vi "niRFUtil WFM Trace Detector.vi"(0 "Real Waveform In (dBm)":T4 {"y" min=0 max=127 format="%.2f"; "dx" format="%^.2e"; "x0" format="%^.2e"}, 5 "Number of Points":T1=1001, 7 "Detector Type":T6=enum."Peak", 11 "error in (no error)":errorcluster, 12 "Averaging Enabled":T3, 13 "Averaging Type":T2) -> (4 "Real Waveform Out (dBm)":T4 {"y" min=0 max=127 format="%.2f"; "dx" format="%^.2e"; "x0" format="%^.2e"}, 6 "Bins per Bucket":i32[](array[numeric]), 15 "error out":errorcluster)   [LabVIEW 2015, in "niRFUtil.lvlib"]
uses:
  niRFUtil.lvlib
  Includes/niRFUtil INC Detector Type.ctl
  Includes/niRFUtil INC Real Waveform.ctl
  Includes/niRFUtil INC Real Array.ctl
  Includes/niRFUtil INC Averaging Enabled.ctl
  Includes/niRFUtil INC Averaging Type (Freq Domain).ctl
  Includes/niRFUtil INC Detector Points.ctl
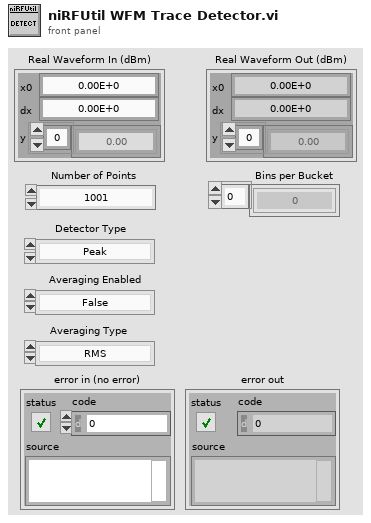
[diagram p1: front panel]
types:
  T1 = typedef "niRFUtil.lvlib/niRFUtil INC Detector Points.ctl" = i32
  T2 = typedef "niRFUtil.lvlib/niRFUtil INC Averaging Type (Freq Domain).ctl" = enum16{"RMS", "Log", "Scalar", "Max", "Min", "Vector"}
  T3 = typedef "niRFUtil.lvlib/niRFUtil INC Averaging Enabled.ctl" = enum16{"False", "True"}
  T4 = typedef "niRFUtil.lvlib/niRFUtil INC Real Waveform.ctl" = cluster{"x0":dbl, "dx":dbl, "y":T5}
  T5 = typedef "niRFUtil.lvlib/niRFUtil INC Real Array.ctl" = sgl[]
  T6 = typedef "niRFUtil.lvlib/niRFUtil INC Detector Type.ctl" = enum16{"Sample", "Normal", "Peak", "Negative Peak", "Average RMS", "Average Voltage", "Average Log"}
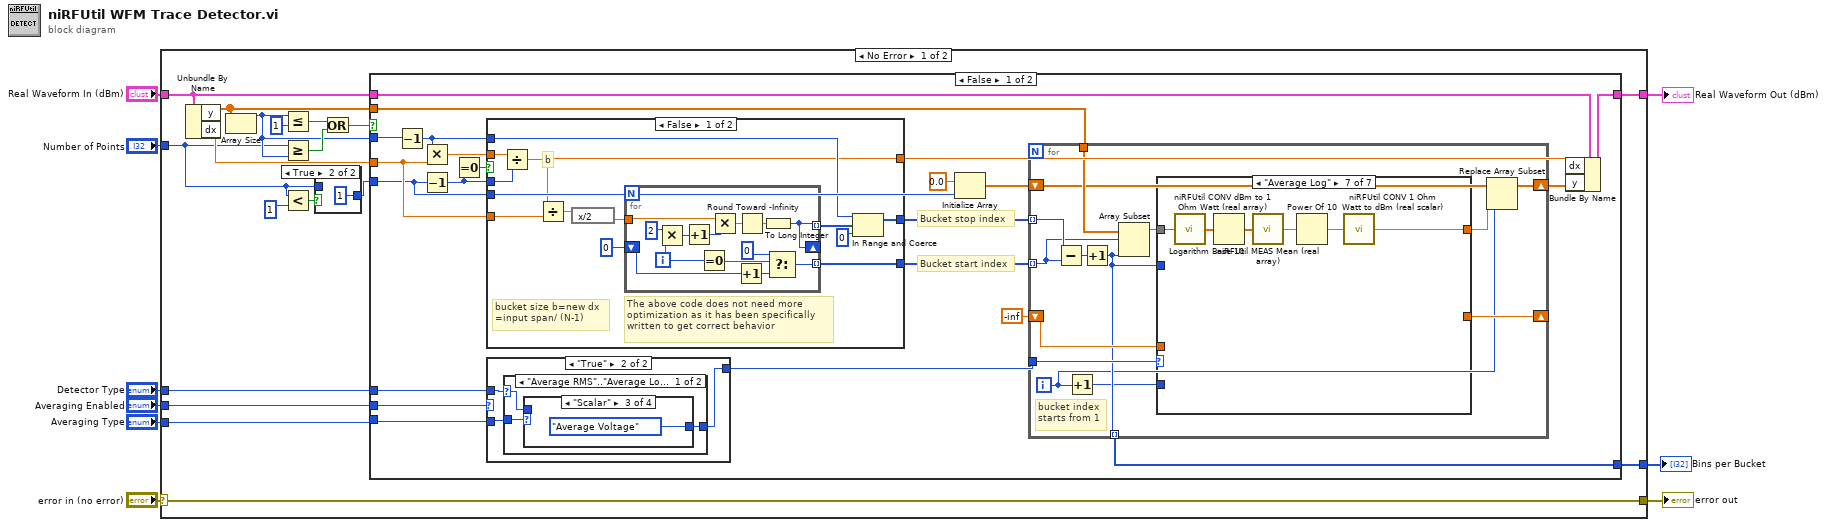
[diagram p0: block diagram]
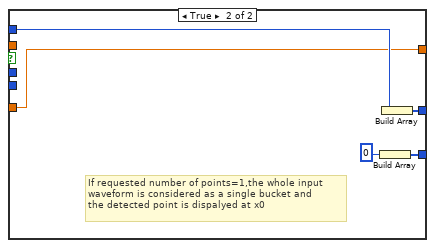
[diagram p3: hidden frame]
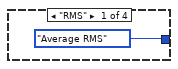
[diagram p5: hidden frame]
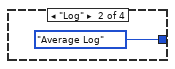
[diagram p6: hidden frame]
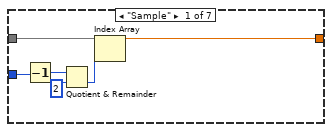
[diagram p9: hidden frame]
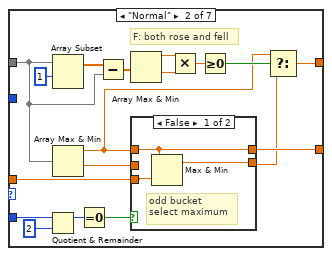
[diagram p10: hidden frame]
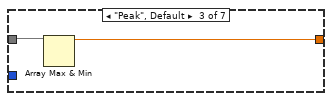
[diagram p12: hidden frame]
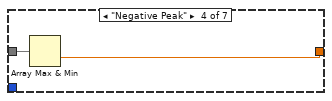
[diagram p13: hidden frame]
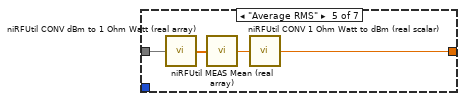
[diagram p14: hidden frame]
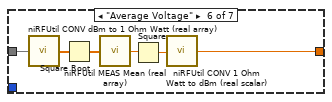
[diagram p15: hidden frame]
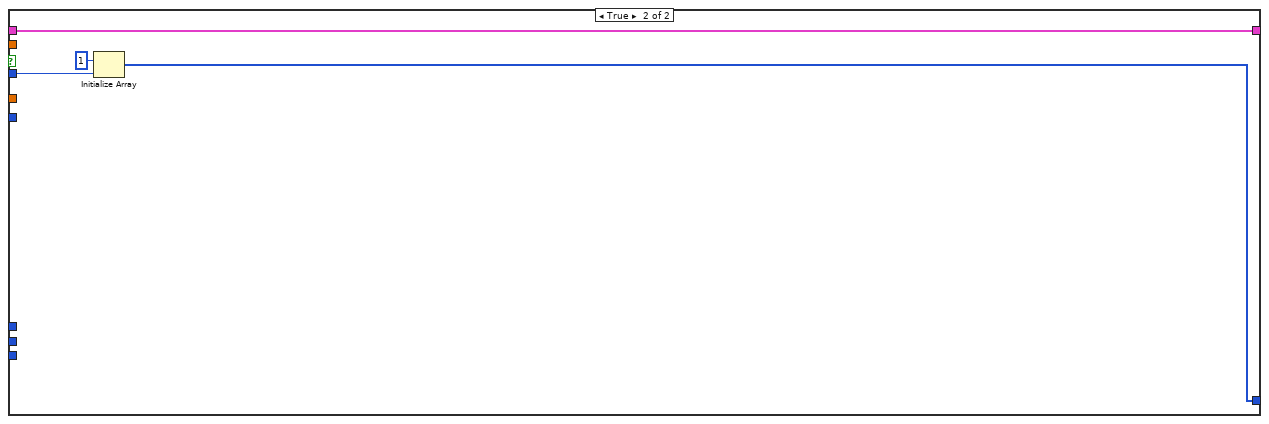
[diagram p16: hidden frame]
diagram:
  n1 = case shown="No Error" "error in (no error)" {
    selector: "error in (no error)" -> [w21 w161]
    tunnel: "Detector Type" -> [w27 _]
    tunnel: "Number of Points" -> [w10 _]
    tunnel: [w26 _] -> w8
    tunnel: [w25 w162] -> w7
    tunnel: "Real Waveform In (dBm)" -> [w24 w162]
    tunnel: "Averaging Enabled" -> [w23 _]
    tunnel: "Averaging Type" -> [w22 _]
    tunnel: [w21 w161] -> w2
    frame No Error {
      n2 = Unbundle By Name(w24) -> ("y"=w19:T5, "dx"=w20:dbl)
      n3 = Array Size(array=w19) -> (size(s)=w14:i32)
      n4 = Less Or Equal?(x=w14, y=1) -> (x <= y?=w17:bool)
      n5 = Greater Or Equal?(x=w10, y=w14) -> (x >= y?=w15:bool)
      n6 = Less?(x=w10, y=T1 1) -> (x < y?=w12:bool)
      n7 = case shown="True" w12 {
        tunnel: w10 -> [w28 _]
        tunnel: [w28 T1 1 ("Number of Points")] -> w11
        frame False {
        }
        frame True {
        }
      }
      n8 = Or(x=w17, y=w15) -> (x .or. y?=w16:bool)
      n9 = case shown="False" w16 {
        tunnel: w27 -> [w39 _]
        tunnel: [w49 w160] -> w25
        tunnel: w20 -> [w42 _]
        tunnel: [w46 w157] -> w26
        tunnel: w24 -> [w44 w160]
        tunnel: w19 -> [w45 _]
        tunnel: w14 -> [w41 w158]
        tunnel: w23 -> [w38 _]
        tunnel: w22 -> [w37 _]
        tunnel: w11 -> [w30 _]
        frame False {
          # "Bucket start index"
          # "Bucket stop index"
          n10 = Decrement(x=w41) -> (x-1=w43:i32)
          n11 = Multiply(x=w43, y=w42) -> (x*y=w51:dbl)
          n12 = Decrement(x=w30) -> (x-1=w32:T1)
          n13 = Equal To 0?(x=w32) -> (x = 0?=w33:bool)
          n14 = case shown="False" w33 {
            tunnel: w51 -> [w64 _]
            tunnel: [w62 w81] -> w48
            tunnel: [w61 w78] -> w47
            tunnel: w43 -> [w56 w82]
            tunnel: w42 -> [w55 w80]
            tunnel: [w54 w80] -> w40
            tunnel: w32 -> [w52 _]
            tunnel: w30 -> [w53 _]
            frame False {
              # "The above code does not need more \noptimization as it has been specifically \nwritten to get correct behavior"
              # "b"
              # "bucket size b=new dx\n=input span/ (N-1)"
              n15 = Divide(x=w64, y=w52) -> (x/y=w54:dbl)
              n16 = Divide(x=w54, y=w55) -> (x/y=w59:dbl)
              n17 = expression code="x/2"(w59) -> (w58:dbl)
              n18 = for {
                N: w53 -> [_]
                tunnel: w58 -> [w74]
                shift-right: [w65] -> _
                shift-left: 0 -> [w69]
                tunnel: [w67] -> w61 mode=indexing
                tunnel: [w65] -> w63 mode=indexing
                i -> [w72]
                n19 = Multiply(x=2 ("y"), y=w72) -> (x*y=w76:i32)
                n20 = Increment(x=w76) -> (x+1=w75:i32)
                n21 = Equal To 0?(x=w72) -> (x = 0?=w71:bool)
                n22 = Multiply(x=w74, y=w75) -> (x*y=w73:dbl)
                n23 = Increment(x=w69) -> (x+1=w68:i32)
                n24 = Round Toward -Infinity(1:w73) -> (0:w66:dbl)
                n25 = To Long Integer(number=w66) -> (32bit integer=w65:i32)
                n26 = Select(t=0 ("y"), s=w71, f=w68) -> (s? t:f=w67:i32)
              }
              n27 = In Range and Coerce(upper limit=w56, x=w63, lower limit=0) -> (coerced(x)=w62:i32[])  [unwired: 1 out]
            }
            frame True {
              # "If requested number of points=1,the whole input\nwaveform is considered as a single bucket and \nthe detected point is dispalyed at x0"
              n28 = Build Array(0 ("y")) -> (w78:i32[])
              n29 = Build Array(w82) -> (w81:i32[])
            }
          }
          n30 = case shown="\"True\"" w38 {
            tunnel: w39 -> [w83 w86]
            tunnel: [w83 w85] -> w36
            tunnel: w37 -> [_ w84]
            frame "False", Default {
            }
            frame "True" {
              n31 = case shown="\"Average RMS\"..\"Average Log\"" w86 {
                selector: w86 -> [w87 w94]
                tunnel: [w88 w94] -> w85
                tunnel: w84 -> [w89 _]
                frame "Average RMS".."Average Log" {
                  n32 = case shown="\"Scalar\"" w89 {
                    tunnel: [niRFUtil_INC_Detector_Type."Average RMS" ("Detector Type") niRFUtil_INC_Detector_Type."Average Log" ("Detector Type") niRFUtil_INC_Detector_Type."Average Voltage" ("Detector Type") w93] -> w88
                    tunnel: w87 -> [_ _ _ w93]
                    frame "RMS" {
                    }
                    frame "Log" {
                    }
                    frame "Scalar" {
                    }
                    frame Default {
                    }
                  }
                }
                frame Default {
                }
              }
            }
          }
          n33 = Initialize Array(sgl 0.0 ("element"), w30) -> (w34:sgl[])
          n34 = for {
            tunnel: w45 -> [w108]
            tunnel: w47 -> [w106] mode=indexing
            tunnel: w48 -> [w107] mode=indexing
            tunnel: w36 -> [w104]
            shift-right: [w95] -> w35
            shift-left: w34 -> [w96]
            shift-right: [w102] -> _
            shift-left: sgl -inf -> [w101]
            tunnel: [w100] -> w46 mode=indexing
            i -> [w98]
            # "bucket index\nstarts from 1"
            n35 = Subtract(x=w107, y=w106) -> (x-y=w105:i32)
            n36 = Increment(x=w98) -> (x+1=w99:i32)
            n37 = Increment(x=w105) -> (x+1=w100:i32)
            n38 = Array Subset(array=w108, index=w106, length=w100) -> (w103:T5)
            n39 = case shown="\"Average Log\"" w104 {
              tunnel: w103 -> [w114 w116 w139 w141 w145 w150 w156]
              tunnel: [w113 w130 w138 w140 w144 w147 w151] -> w97
              tunnel: w99 -> [_ w129 _ _ _ _ _]
              tunnel: [_ w126 _ _ _ _ _] -> w102
              tunnel: w101 -> [_ w125 _ _ _ _ _]
              tunnel: w100 -> [w109 _ _ _ _ _ _]
              frame "Sample" {
                n40 = Decrement(x=w109) -> (x-1=w112:i32)
                n41 = Quotient & Remainder(x=w112, y=2) -> (floor(x/y)=w110:i32)  [unwired: 1 out]
                n42 = Index Array(array=w114, index=w110) -> (element=w113:sgl)
              }
              frame "Normal" {
                # "F: both rose and fell"
                n43 = Quotient & Remainder(x=w129, y=2) -> (x-y*floor(x/y)=w127:i32)  [unwired: 1 out]
                n44 = Array Subset(array=w116, index=1) -> (w117:T5)  [unwired: 1 in]
                n45 = Array Max & Min(array=w116) -> (max value=w119:sgl, min value=w118:sgl)  [unwired: 2 out]
                n46 = Equal To 0?(x=w127) -> (x = 0?=w115:bool)
                n47 = Subtract(x=w117, y=w116) -> (x-y=w131:T5)
                n48 = Array Max & Min(array=w131) -> (max value=w124:sgl, min value=w123:sgl)  [unwired: 2 out]
                n49 = case shown="False" w115 {
                  tunnel: [w134 w136] -> w120
                  tunnel: [w133 w137] -> w126
                  tunnel: w125 -> [w135 _]
                  tunnel: w119 -> [w133 w137]
                  tunnel: w118 -> [_ w136]
                  frame False {
                    # "odd bucket \nselect maximum"
                    n50 = Max & Min(x=w133, y=w135) -> (max(x,y)=w134:sgl)  [unwired: 1 out]
                  }
                  frame True {
                    # "even bucket \nselect minimum"
                  }
                }
                n51 = Multiply(x=w124, y=w123) -> (x*y=w122:sgl)
                n52 = Greater Or Equal To 0?(x=w122) -> (x >= 0?=w121:bool)
                n53 = Select(t=w119, s=w121, f=w120) -> (s? t:f=w130:sgl)
              }
              frame "Peak", Default {
                n54 = Array Max & Min(array=w139) -> (max value=w138:sgl)  [unwired: 3 out]
              }
              frame "Negative Peak" {
                n55 = Array Max & Min(array=w141) -> (min value=w140:sgl)  [unwired: 3 out]
              }
              frame "Average RMS" {
                n56 = call "niRFUtil CONV dBm to 1 Ohm Watt (real array).vi"("Real Array (dBm)"=w145) -> ("Real Array (W)"=w143:T5)  [unwired: 14 in]
                n57 = call "niRFUtil MEAS Mean (real array).vi"("Real Array"=w143) -> ("Mean"=w142:sgl)  [unwired: 14 in]
                n58 = call "niRFUtil CONV 1 Ohm Watt to dBm (real scalar).vi"("Real Scalar (W)"=w142) -> ("Real Scalar (dBm)"=w144:sgl)  [unwired: 14 in]
              }
              frame "Average Voltage" {
                n59 = call "niRFUtil CONV dBm to 1 Ohm Watt (real array).vi"("Real Array (dBm)"=w150) -> ("Real Array (W)"=w149:T5)  [unwired: 14 in]
                n60 = Square Root(x=w149) -> ()  [unwired: 1 out]
                n61 = call "niRFUtil MEAS Mean (real array).vi"("Real Array"=w149) -> ("Mean"=w146:sgl)  [unwired: 14 in]
                n62 = Square(x=w146) -> (x^2=w148:sgl)
                n63 = call "niRFUtil CONV 1 Ohm Watt to dBm (real scalar).vi"("Real Scalar (W)"=w148) -> ("Real Scalar (dBm)"=w147:sgl)  [unwired: 14 in]
              }
              frame "Average Log" {
                n64 = call "niRFUtil CONV dBm to 1 Ohm Watt (real array).vi"("Real Array (dBm)"=w156) -> ("Real Array (W)"=w155:T5)  [unwired: 14 in]
                n65 = Logarithm Base 10(1:w155) -> (0:w154:T5)
                n66 = call "niRFUtil MEAS Mean (real array).vi"("Real Array"=w154) -> ("Mean"=w153:sgl)  [unwired: 14 in]
                n67 = Power Of 10(x=w153) -> (10^x=w152:sgl)
                n68 = call "niRFUtil CONV 1 Ohm Watt to dBm (real scalar).vi"("Real Scalar (W)"=w152) -> ("Real Scalar (dBm)"=w151:sgl)  [unwired: 14 in]
              }
            }
            n69 = Replace Array Subset(array=w96, new element=w97, index=w98) -> (w95:sgl[])
          }
          n70 = Bundle By Name(cluster=w44, "dx"=w40, "y"=w35) -> (w49:T4)
        }
        frame True {
          n71 = Initialize Array(1 ("element"), w158) -> (w157:i32[])
        }
      }
    }
    frame Error {
    }
  }
  "Real Waveform Out (dBm)" <- w7
  "Bins per Bucket" <- w8
  "error out" <- w2
